vi "Amp_PS_onoff - Copy.vi"(2 "error in (no error)":errorcluster, 3 "On/Off Control":string(combo), 4 "delay before read (ms)":u32=500, 5 "Amp PS address":refnum<visa-resource-name>) -> (0 "error out":errorcluster, 1 "status":bool)   [LabVIEW 2013]
panel:
  out "return count":u32
  out "read buffer":string
  out "Serial Settings:Number of Bytes at Serial Port":u32
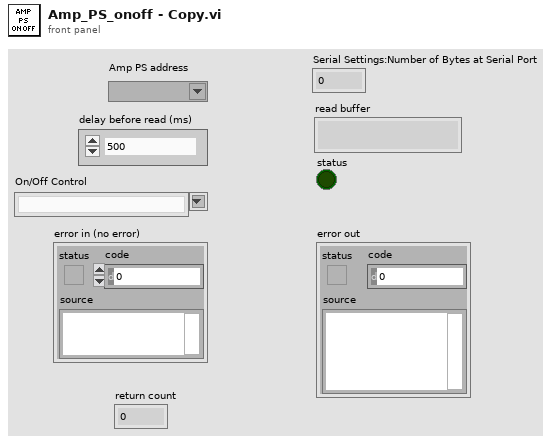
[diagram p1: front panel]
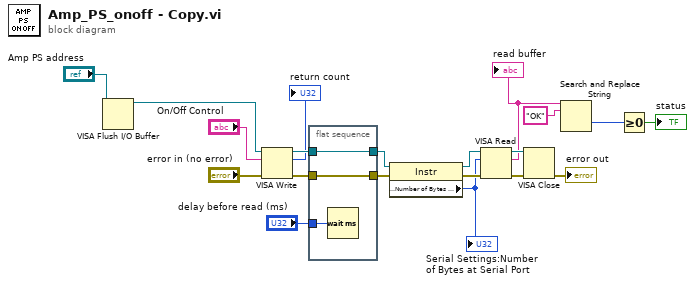
[diagram p0: block diagram]
diagram:
  n1 = VISA Flush I/O Buffer(VISA resource name="Amp PS address") -> (VISA resource name out=w1:refnum<visa-resource-name>)  [unwired: 2 in, 1 out]
  n2 = VISA Write(VISA resource name=w1, write buffer="On/Off Control", error in (no error)="error in (no error)") -> (VISA resource name out=w16:refnum<visa-resource-name>, return count=→"return count":u32, error out=w18:errorcluster)
  n3 = flat-sequence {
    tunnel: w18 -> [w22]
    tunnel: [w22] -> w17
    tunnel: w16 -> [w21]
    tunnel: [w21] -> w15
    tunnel: "delay before read (ms)" -> [w23]
    frame #0 {
      n4 = Wait (ms)(milliseconds to wait=w23) -> ()  [unwired: 1 out]
    }
  }
  n5 = property class="Instr"(reference=w15, error in=w17) -> (reference out=w14:refnum<visa-resource-name>, error out=w13:errorcluster, "Serial Settings:Number of Bytes at Serial Port"=w12:u32)
  "Serial Settings:Number of Bytes at Serial Port" <- w12
  n6 = VISA Read(VISA resource name=w14, byte count=w12, error in (no error)=w13) -> (VISA resource name out=w19:refnum<visa-resource-name>, read buffer=w8:string, error out=w20:errorcluster)  [unwired: 1 out]
  "read buffer" <- w8
  n7 = VISA Close(VISA resource name=w19, error in (no error)=w20) -> (error out=→"error out":errorcluster)
  n8 = Search and Replace String(input string=w8, search string="OK" ("true string")) -> (offset past replacement=w6:i32)  [unwired: 6 in, 3 out]
  n9 = Greater Or Equal To 0?(x=w6) -> (x >= 0?=→"status":bool)
